vi "PacMan Test 2.vi"() -> ()   [LabVIEW 2016]
uses:
  PacMan Classes/Generic Controls/Picture.ctl
  PacMan Classes/Generic Controls/Direction.ctl
  PacMan Classes/Circle/PacMan.lvclass
  C:/Users/lucamach/Documents/SE/Learning OOP/PacMan/PacMan Classes/Geometric Figure/UI Object.lvclass
  PacMan Classes/Generic Controls/Pen.ctl
  PacMan Classes/Generic Controls/Point.ctl
  PacMan Classes/Generic Controls/Color.ctl
  PacMan Classes/Geometric Figure/UI Object.lvclass/UI Object.ctl
  PacMan Classes/Geometric Figure/Write Color (RGB).vi
  PacMan Classes/Geometric Figure/Write Center (px).vi
  PacMan Classes/PacManClasses.lvlib
panel:
  in  "Move Data 2":cluster{"Direction":T1, "Step (px)":u16}
  in  "Move Data":cluster{"Direction":T1, "Step (px)":u16}
  out "Picture":T2
  in  "stop":bool
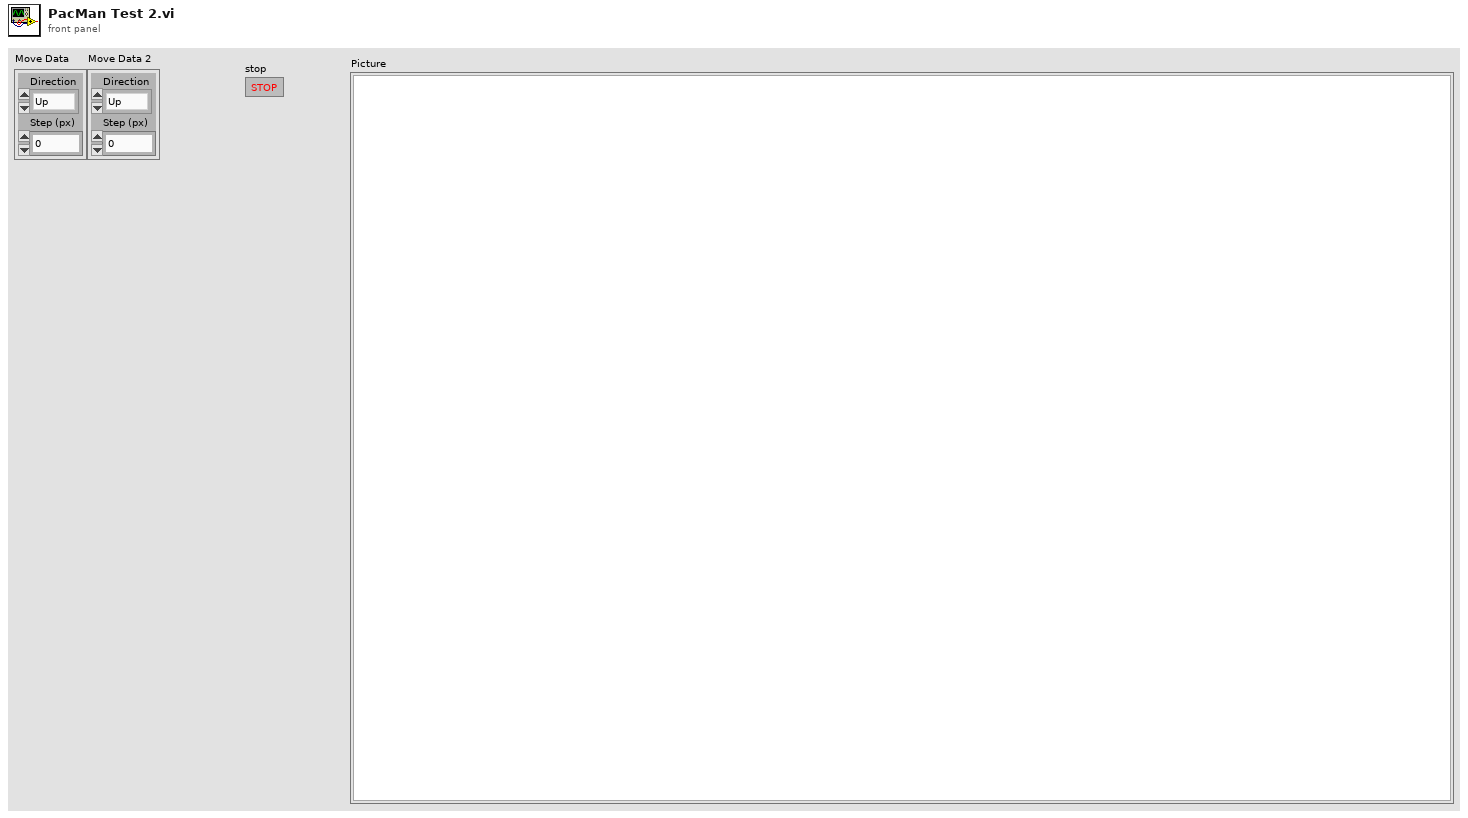
[diagram p1: front panel]
types:
  T1 = typedef "PacManClasses.lvlib/Direction.ctl" = enum16{"Up", "Down", "Left", "Right"}
  T2 = typedef "PacManClasses.lvlib/Picture.ctl" = picture
  T3 = typedef "PacManClasses.lvlib/Color.ctl" = cluster{"Red":u8, "Green":u8, "Blue":u8}
  T4 = typedef "PacManClasses.lvlib/Point.ctl" = cluster{"x":u16, "y":u16}
  T5 = typedef "PacManClasses.lvlib/Pen.ctl" = cluster{"Width":u16, "Style":enum32{"Solid", "Dash", "Dot", "DashDot", "DashDotDot"}}
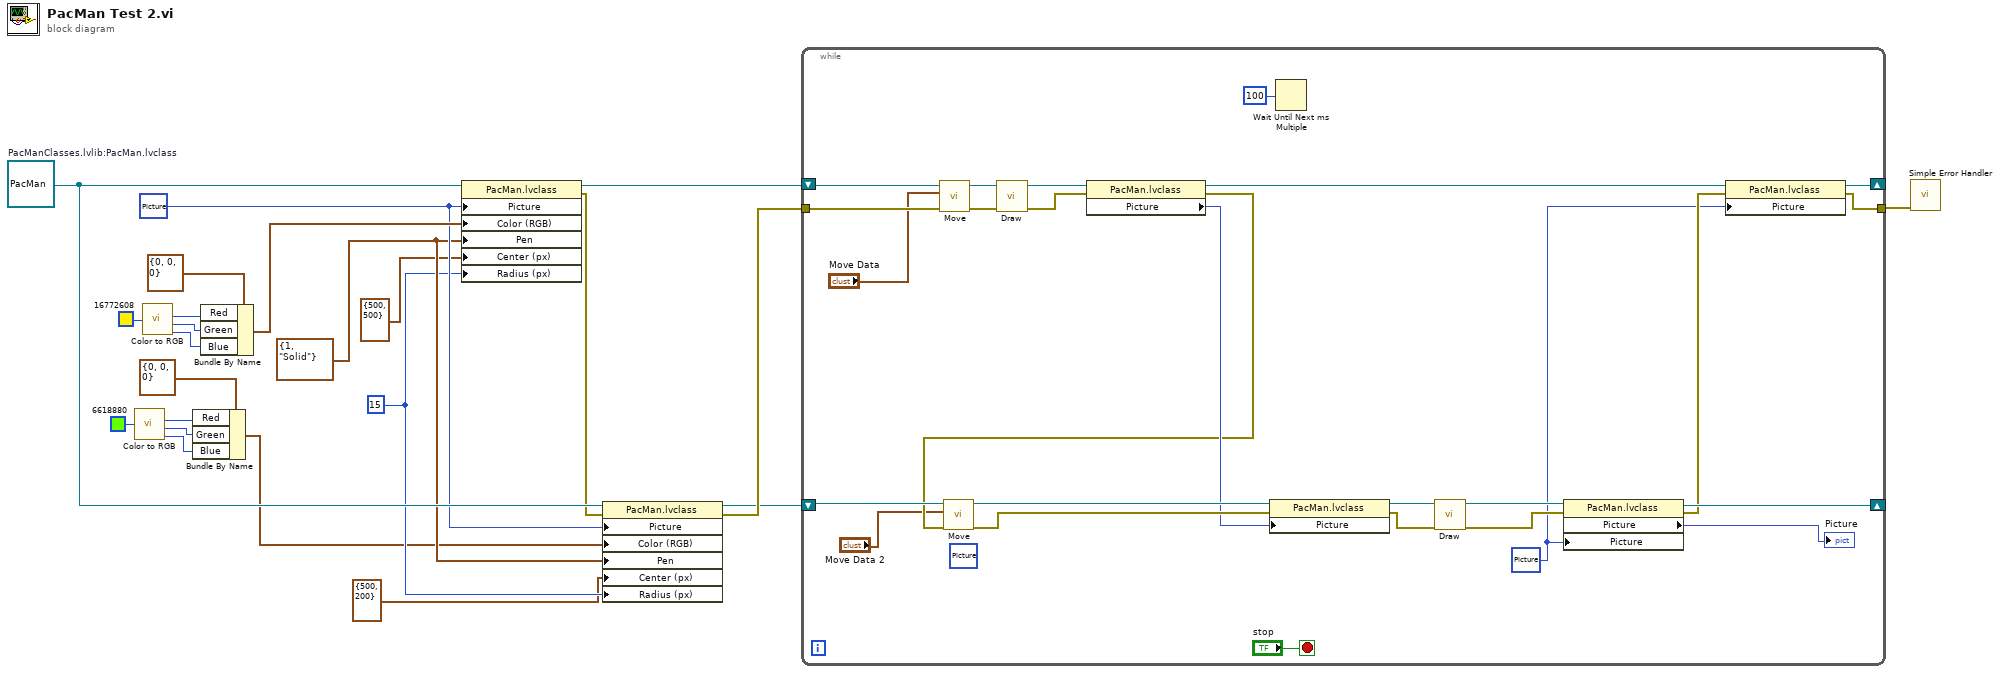
[diagram p0: block diagram]
diagram:
  w13 = T5 {"Width"=1, "Style"=enum."Solid"} ("pen")
  w14 = T2 data[5B] ("Picture")
  w16 = refnum<class "PacMan.lvclass"> refnum  # PacManClasses.lvlib:PacMan.lvclass
  w11 = u16 15 ("Radius (px)")
  n1 = call <vilib>:"Color to RGB.vi"("Color"=u32 6618880) -> ("R"=w4:u8, "G"=w5:u8, "B"=w6:u8)  [unwired: 1 out]
  n2 = call <vilib>:"Color to RGB.vi"("Color"=u32 16772608) -> ("R"=w21:u8, "G"=w20:u8, "B"=w19:u8)  [unwired: 1 out]
  n3 = Bundle By Name(cluster=T3 {"Red"=0, "Green"=0, "Blue"=0} ("Color (RGB)"), "Red"=w4, "Green"=w5, "Blue"=w6) -> (w1:T3)
  n4 = Bundle By Name(cluster=T3 {"Red"=0, "Green"=0, "Blue"=0} ("Color (RGB)"), "Red"=w21, "Green"=w20, "Blue"=w19) -> (w15:T3)
  n5 = property class="PacMan.lvclass"(reference=w16, "Picture"=w14, "Color (RGB)"=w15, "Pen"=w13, "Center (px)"=T4 {"x"=500, "y"=500} ("Point (px)"), "Radius (px)"=w11) -> (reference out=w18:refnum<class "PacMan.lvclass">, error out=w10:errorcluster)  [unwired: 1 in]
  n6 = property class="PacMan.lvclass"(reference=w16, error in=w10, "Picture"=w14, "Color (RGB)"=w1, "Pen"=w13, "Center (px)"=T4 {"x"=500, "y"=200} ("Point (px)"), "Radius (px)"=w11) -> (reference out=w8:refnum<class "PacMan.lvclass">, error out=w9:errorcluster)
  n7 = while {
    tunnel: [w24] -> w23
    tunnel: w9 -> [w46]
    shift-right: [w27] -> _
    shift-left: w18 -> [w47]
    shift-right: [w29] -> _
    shift-left: w8 -> [w38]
    stop <- "stop" stop-if-true
    w25 = T2 data[5B] ("Picture")
    (unwired) T2 data[5B] ("Picture")
    n8 = call-dynamic "Move.vi"("error in (no error)"=w46, "Move Data"="Move Data", "PacMan In"=w47) -> ("error out"=w44:errorcluster, "PacMan Out"=w45:refnum<class "PacMan.lvclass">)  [unwired: 7 in]
    n9 = call-dynamic "Draw.vi"("error in (no error)"=w44, "Circle in"=w45) -> ("error out"=w43:errorcluster, "Circle out"=w42:refnum<class "PacMan.lvclass">)  [unwired: 8 in]
    n10 = property class="PacMan.lvclass"(reference=w42, error in=w43) -> (reference out=w28:refnum<class "PacMan.lvclass">, error out=w32:errorcluster, "Picture"=w33:T2)
    n11 = call-dynamic "Move.vi"("error in (no error)"=w32, "Move Data"="Move Data 2", "PacMan In"=w38) -> ("error out"=w36:errorcluster, "PacMan Out"=w37:refnum<class "PacMan.lvclass">)  [unwired: 7 in]
    n12 = property class="PacMan.lvclass"(reference=w37, error in=w36, "Picture"=w33) -> (reference out=w35:refnum<class "PacMan.lvclass">, error out=w34:errorcluster)
    n13 = Wait Until Next ms Multiple(millisecond multiple=u32 100) -> ()  [unwired: 1 out]
    n14 = call-dynamic "Draw.vi"("error in (no error)"=w34, "Circle in"=w35) -> ("error out"=w39:errorcluster, "Circle out"=w40:refnum<class "PacMan.lvclass">)  [unwired: 8 in]
    n15 = property class="PacMan.lvclass"(reference=w40, error in=w39, "Picture"=w25) -> (reference out=w29:refnum<class "PacMan.lvclass">, error out=w26:errorcluster, "Picture"=→"Picture":T2)
    n16 = property class="PacMan.lvclass"(reference=w28, error in=w26, "Picture"=w25) -> (reference out=w27:refnum<class "PacMan.lvclass">, error out=w24:errorcluster)
  }
  n17 = call <vilib>:"Simple Error Handler.vi"("error in (no error)"=w23) -> ()  [unwired: 4 in, 5 out]
